vi "Actor Core.vi"(8 "error in":errorcluster, 11 "Car Wash Display ViewManager In":refnum<class "Car Wash Display ViewManager.lvclass">) -> (0 "error out":errorcluster, 3 "Actor out":refnum<class "Actor.lvclass">)   [LabVIEW 2019, in "Car Wash Display ViewManager.lvclass"]
doc: "(<B>Filename</B>: Actor Framework.lvlib:Actor.lvclass:Actor Core.vi)\n\nReceives messages to the actor, reacts to them, and initiates any error handling that may shut the actor down.\n\nDescendant classes may override this VI to append parallel tasks for the actor to complete while it handles messages. Overrides use the Call Parent Method node.\n\n<License>\nCopyright © 2017 Composed Systems, LLC | All rights reserved\nwww.composed.io\n\nAuthor: Ethan Stern <ethan.stern@composed.io>\n\nThis software is provided \"AS IS\" WITHOUT WARRANTIES, either express or implied, AND IS FOR EDUCATIONAL PURPOSES ONLY.\n</License>"
uses:
  <vilib>/gpm_packages/@cs/Car-wash/Source/Car Wash Display ViewManager/Car Wash Display ViewManager/Car Wash Display ViewManager.lvclass
  <vilib>/gpm_packages/@cs/mva-viewable/Source/IViewable/ProtectedSubpanel/ProtectedSubpanel.lvclass
  <vilib>/gpm_packages/@cs/mva-viewable/Source/IViewManager/IViewManager/IViewManager.lvclass
  <vilib>/ActorFramework/Actor/Actor.lvclass
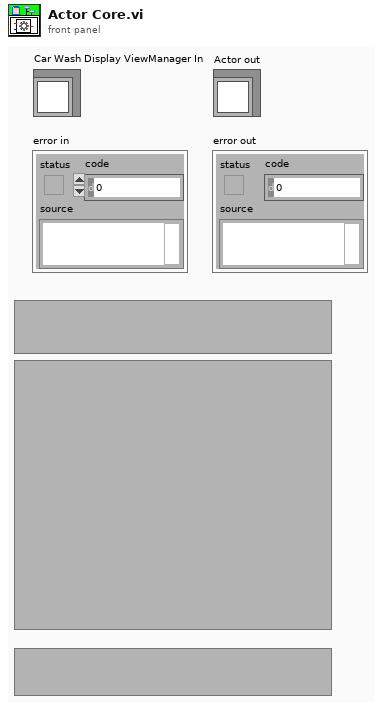
[diagram p1: front panel]
types:
  T1 = typedef "IViewable.lvlib/ProtectedSubpanel.lvclass/Protected Subpanel Reference.ctl" = refnum<data-value>
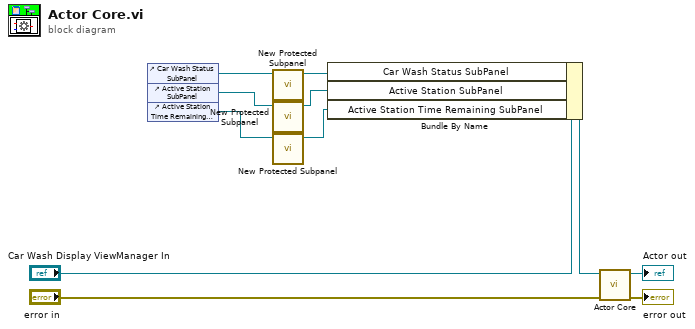
[diagram p0: block diagram]
diagram:
  n1 = control-ref of="Car Wash Status SubPanel"() -> (w8:refnum<vi>)
  n2 = control-ref of="Active Station SubPanel"() -> (w7:refnum<vi>)
  n3 = control-ref of="Active Station Time Remaining SubPanel"() -> (w6:refnum<vi>)
  n4 = call <vilib>:"New Protected Subpanel.vi"("SubPnl Refnum"=w8) -> ("Protected Subpanel"=w3:T1)  [unwired: 9 in, 1 out]
  n5 = call <vilib>:"New Protected Subpanel.vi"("SubPnl Refnum"=w7) -> ("Protected Subpanel"=w2:T1)  [unwired: 9 in, 1 out]
  n6 = call <vilib>:"New Protected Subpanel.vi"("SubPnl Refnum"=w6) -> ("Protected Subpanel"=w1:T1)  [unwired: 9 in, 1 out]
  n7 = Bundle By Name(cluster="Car Wash Display ViewManager In", "Car Wash Status SubPanel"=w3, "Active Station SubPanel"=w2, "Active Station Time Remaining SubPanel"=w1) -> (w4:refnum<class "Car Wash Display ViewManager.lvclass">)
  n8 = call-parent "Actor Core.vi"("error in"="error in", "IViewable In"=w4) -> ("error out"=→"error out":errorcluster, "Actor out"=→"Actor out":refnum<class "Actor.lvclass">)  [unwired: 8 in]
